vi "solar_misc xml Escape.vi"(0 "XML in":string, 1 "Action (Escape)":enum8{"Escape", "Unescape"}(ring)) -> (6 "XML out":string)   [LabVIEW 2018]
doc: "This VI escapes or unescapes xml characters including decimals 128 to 255.\n\" = &quot;\n' = &apos;\n< = &lt;\n> = &gt;\n& = &amp;"
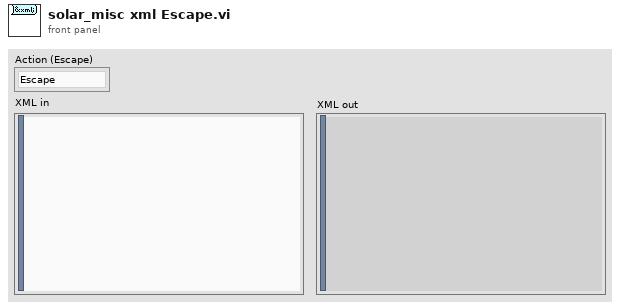
[diagram p1: front panel]
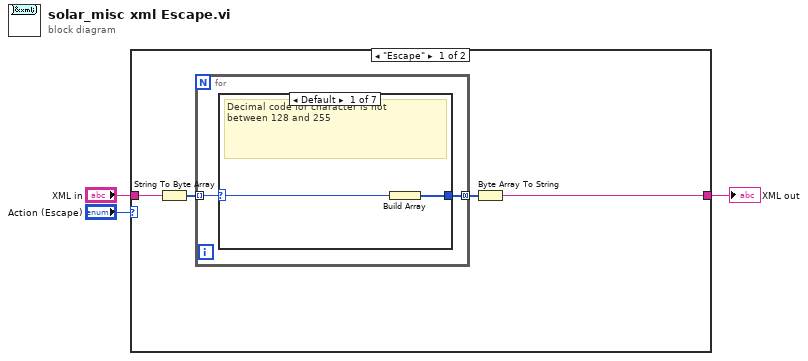
[diagram p0: block diagram]
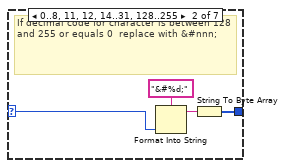
[diagram p2: hidden frame]
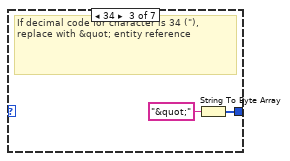
[diagram p3: hidden frame]
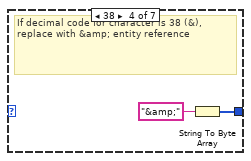
[diagram p4: hidden frame]
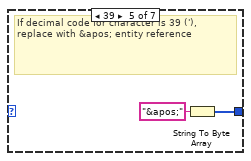
[diagram p5: hidden frame]
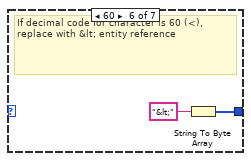
[diagram p6: hidden frame]
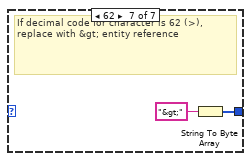
[diagram p7: hidden frame]
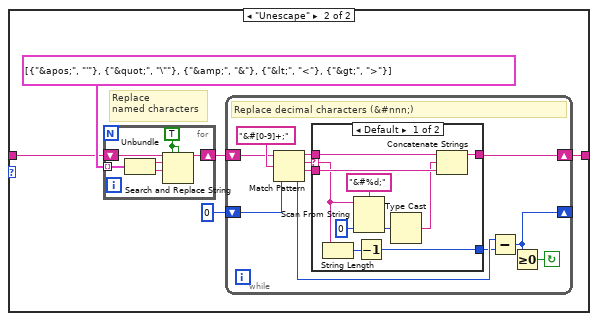
[diagram p8: hidden frame]
diagram:
  n1 = case shown="\"Escape\"" "Action (Escape)" {
    tunnel: "XML in" -> [w5 w27]
    tunnel: [w4 w26] -> w1
    frame "Escape" {
      n2 = String To Byte Array(string=w5) -> (unsigned byte array=w7:u8[])
      n3 = for {
        tunnel: w7 -> [w8] mode=indexing
        tunnel: [w9] -> w6 mode=concatenating
        n4 = case shown="Default" w8 {
          selector: w8 -> [w10 w13 _ _ _ _ _]
          tunnel: [w11 w12 w16 w18 w20 w22 w24] -> w9
          frame Default {
            # "Decimal code for character is not \nbetween 128 and 255"
            n5 = Build Array(w10) -> (w11:u8[])
          }
          frame 0..8, 11, 12, 14..31, 128..255 {
            # "If decimal code for character is between 128 and 255 or equals 0  replace with &#nnn;"
            n6 = Format Into String(format string="&#%d;" ("Format String"), w13) -> (resulting string=w14:string)  [unwired: 2 in, 1 out]
            n7 = String To Byte Array(string=w14) -> (unsigned byte array=w12:u8[])
          }
          frame 34 {
            # "If decimal code for character is 34 (\"),\nreplace with &quot; entity reference"
            n8 = String To Byte Array(string="&quot;" ("Format String")) -> (unsigned byte array=w16:u8[])
          }
          frame 38 {
            # "If decimal code for character is 38 (&),\nreplace with &amp; entity reference"
            n9 = String To Byte Array(string="&amp;" ("Format String")) -> (unsigned byte array=w18:u8[])
          }
          frame 39 {
            # "If decimal code for character is 39 ('),\nreplace with &apos; entity reference"
            n10 = String To Byte Array(string="&apos;" ("Format String")) -> (unsigned byte array=w20:u8[])
          }
          frame 60 {
            # "If decimal code for character is 60 (<),\nreplace with &lt; entity reference"
            n11 = String To Byte Array(string="&lt;" ("Format String")) -> (unsigned byte array=w22:u8[])
          }
          frame 62 {
            # "If decimal code for character is 62 (>),\nreplace with &gt; entity reference"
            n12 = String To Byte Array(string="&gt;" ("Format String")) -> (unsigned byte array=w24:u8[])
          }
        }
      }
      n13 = Byte Array To String(unsigned byte array=w6) -> (string=w4:string)
    }
    frame "Unescape" {
      # "Replace \nnamed characters"
      n14 = for {
        shift-right: [w35] -> w29
        shift-left: w27 -> [w36]
        tunnel: cluster{string, string}[] [{"&apos;", "'"}, {"&quot;", "\""}, {"&amp;", "&"}, {"&lt;", "<"}, {"&gt;", ">"}] -> [w34] mode=indexing
        w31 = TRUE ("replace all? (F)")
        n15 = Unbundle(w34) -> (w33:string, w32:string)
        n16 = Search and Replace String(replace all?=w31, case sensitive?=w31, input string=w36, search string=w33, replace string=w32) -> (result string=w35:string)  [unwired: 3 in, 3 out]
      }
      n17 = while {
        shift-left: 0 -> [w46]
        shift-right: [w39] -> _
        shift-left: w29 -> [w38]
        shift-right: [w42] -> w26
        stop <- w41 continue-if-true
        # "Replace decimal characters (&#nnn;)"
        n18 = Match Pattern(string=w38, regular expression="&#[0-9]+;", offset (0)=w46) -> (before substring=w44:string, match substring=w45:string, after substring=w43:string, offset past match=w40:i32)
        n19 = case shown="Default" w45 {
          selector: w45 -> [w53 _]
          tunnel: w44 -> [w57 w58]
          tunnel: w43 -> [w55 _]
          tunnel: [w56 w58] -> w42
          tunnel: [w48 _] -> w37
          frame Default {
            n20 = String Length(string=w53) -> (length=w49:i32)
            n21 = Scan From String(format string="&#%d;" ("Input String"), input string=w53, default 1=u8 0) -> (output 1=w51:u8)  [unwired: 2 in, 3 out]
            n22 = Decrement(x=w49) -> (x-1=w48:i32)
            n23 = Type Cast(x=w51) -> (*(type *) &x=w50:string)  [unwired: 1 in]
            n24 = Concatenate Strings(w57, w50, w55) -> (w56:string)
          }
          frame "" {
          }
        }
        n25 = Subtract(x=w40, y=w37) -> (x-y=w39:i32)
        n26 = Greater Or Equal To 0?(x=w39) -> (x >= 0?=w41:bool)
      }
    }
  }
  "XML out" <- w1
